vi "dfd_Validate SRate Quantizers for Code Gen.vi"(4 "FPGA?":bool=TRUE, 6 "LabVIEW?":bool=TRUE, 8 "error in (no error)":errorcluster, 11 "filter in":T1={"mSRate_Fs"=1.0, "mSRate_Version"="1.0", "mSRate_Comments"="", "mSRate_OrgCoef"={"type"=enum."Undefined", "gain"=1.0, "coef a (k)"=[], "coef b (v)"=[]}, "mSRate_CurCoef"={"type"=enum."Undefined", "gain"=1.0, "coef a (k)"=[], "coef b (v)"=[]}, "mSRate_Quantized?"=FALSE, "mSRate_QCoef"={"type"=enum."Undefined", "gain"=1.0, "coef a (k)"=[], "coef b (v)"=[]}, "mSRate_QSettings"=[], "mSRate_Order"=0, "mSRate_Scaling"={"mSRate_ScaleByPowerOf2?"=FALSE, "mSRate_ScaleType"=enum."No Norm"}} {"mSRate_QSettings"."source" items=["Coef a/k"=0, "Coef b/v"=7, "Input"=1, "Output"=2, "Multiplicand"=3, "Product"=4, "Sum"=5, "Delay"=6, "Gain"=8]}) -> (0 "error out":errorcluster, 3 "filter out":T1={"mSRate_Fs"=1.0, "mSRate_Version"="1.0", "mSRate_Comments"="", "mSRate_OrgCoef"={"type"=enum."Undefined", "gain"=1.0, "coef a (k)"=[], "coef b (v)"=[]}, "mSRate_CurCoef"={"type"=enum."Undefined", "gain"=1.0, "coef a (k)"=[], "coef b (v)"=[]}, "mSRate_Quantized?"=FALSE, "mSRate_QCoef"={"type"=enum."Undefined", "gain"=1.0, "coef a (k)"=[], "coef b (v)"=[]}, "mSRate_QSettings"=[], "mSRate_Order"=0, "mSRate_Scaling"={"mSRate_ScaleByPowerOf2?"=FALSE, "mSRate_ScaleType"=enum."No Norm"}} {"mSRate_QSettings"."source" items=["Coef a/k"=0, "Coef b/v"=7, "Input"=1, "Output"=2, "Multiplicand"=3, "Product"=4, "Sum"=5, "Delay"=6, "Gain"=8]})   [LabVIEW 2017, in "NI_DigFilterLicensed.lvlib"]
uses:
  <vilib>/addons/Digital Filter Design/NI_DigFilterLicensed.lvlib
  <vilib>/addons/Digital Filter Design/_Objects.llb/DFD Filter Obj.ctl
  <vilib>/addons/Digital Filter Design/_Objects.llb/DFD Filter Coef.ctl
  <vilib>/addons/Digital Filter Design/_Objects.llb/DFD Filter Structure Type Selector.ctl
  <vilib>/addons/Digital Filter Design/_Objects.llb/dfd_Internal Quantization Settings.ctl
  <vilib>/addons/Digital Filter Design/_Objects.llb/dfd_Internal Quantization Srcs.ctl
  <vilib>/addons/Digital Filter Design/_Objects.llb/DFD Coef Norm Type.ctl
  <vilib>/addons/Digital Filter Design/_Misc.llb/dfd_Error Handlers (Multiple).vi
  <vilib>/addons/Digital Filter Design/FilterLib.llb/dfd_Get Filter Coef Type (Filter IO).vi
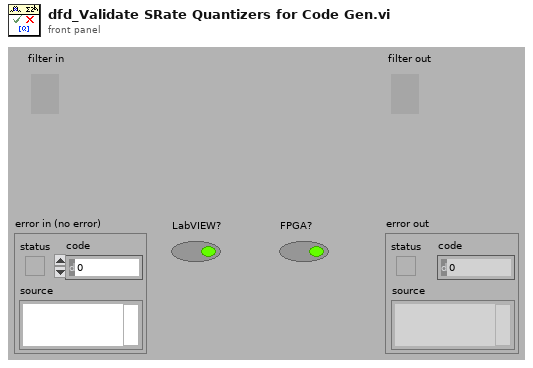
[diagram p1: front panel]
types:
  T1 = typedef "NI_DigFilterLicensed.lvlib/DFD Filter Obj.ctl" = cluster{"mSRate_Fs":dbl, "mSRate_Version":string, "mSRate_Comments":string, "mSRate_OrgCoef":T2, "mSRate_CurCoef":T2, "mSRate_Quantized?":bool, "mSRate_QCoef":T2, "mSRate_QSettings":T4[], "mSRate_Order":i32, "mSRate_Scaling":cluster{"mSRate_ScaleByPowerOf2?":bool, "mSRate_ScaleType":T6}}
  T2 = typedef "NI_DigFilterLicensed.lvlib/DFD Filter Coef.ctl" = cluster{"type":T3, "gain":dbl, "coef a (k)":dbl[], "coef b (v)":dbl[]}
  T3 = typedef "NI_DigFilterLicensed.lvlib/DFD Filter Structure Type Selector.ctl" = enum16{"Undefined", "FIR Direct Form", "FIR Direct Form Transposed", "FIR Symmetric", "FIR Antisymmetric", "IIR Direct Form I", "IIR Direct Form I Transposed", "IIR Direct Form II", "IIR Direct Form II Transposed", "IIR Cascaded Second Order Sections Form I", "IIR Cascaded Second Order Sections Form I Transposed", "IIR Cascaded Second Order Sections Form II", "IIR Cascaded Second Order Sections Form II Transposed", "Lattice Allpass (basic sections)", "Lattice Allpass (one multiplier sections)", "Lattice Allpass (normalized sections)", "Lattice AR (basic sections)", "Lattice AR (one multiplier sections)", "Lattice AR (normalized sections)", "Lattice MA (minimum phase)", "Lattice MA (maximum phase)", "Lattice ARMA (basic sections)", "Lattice ARMA (one multiplier sections)", "Lattice ARMA (normalized sections)"}
  T4 = typedef "NI_DigFilterLicensed.lvlib/dfd_Internal Quantization Settings.ctl" = cluster{"source":T5, "wl":i16, "iwl":i16, "overflow mode":enum16{"Saturation", "Wrap"}, "rounding mode":enum16{"Nearest", "Truncation"}, "signed?":bool}
  T5 = typedef "NI_DigFilterLicensed.lvlib/dfd_Internal Quantization Srcs.ctl" = u16
  T6 = typedef "NI_DigFilterLicensed.lvlib/DFD Coef Norm Type.ctl" = enum16{"No Norm", "Time Domain 1-Norm", "Time Domain 2-Norm", "Time Domain Inf-Norm"}
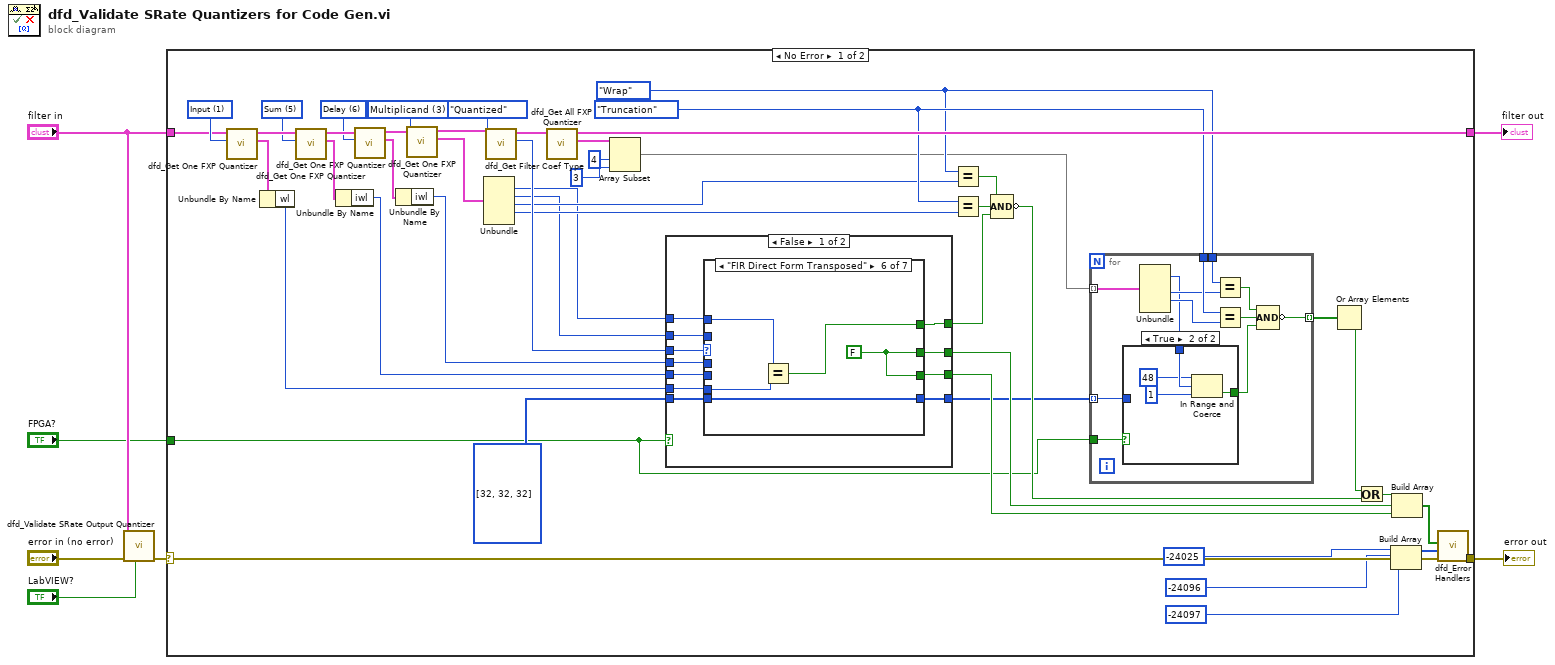
[diagram p0: block diagram]
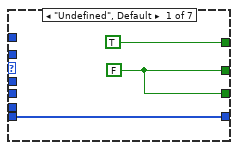
[diagram p2: hidden frame]
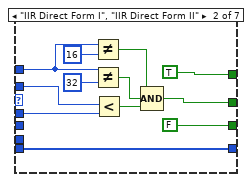
[diagram p3: hidden frame]
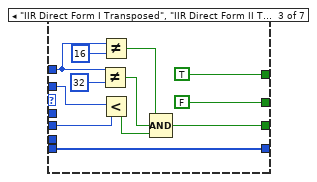
[diagram p4: hidden frame]
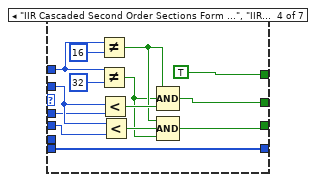
[diagram p5: hidden frame]
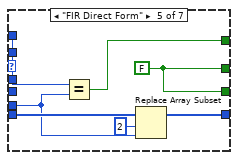
[diagram p6: hidden frame]
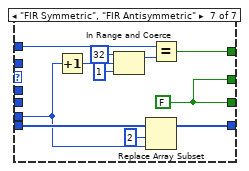
[diagram p7: hidden frame]
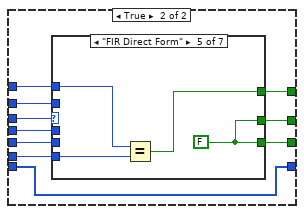
[diagram p8: hidden frame]
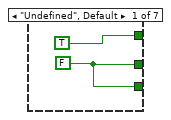
[diagram p9: hidden frame]
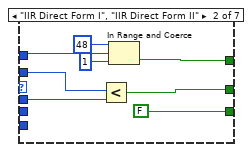
[diagram p10: hidden frame]
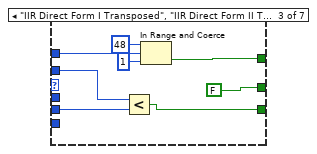
[diagram p11: hidden frame]
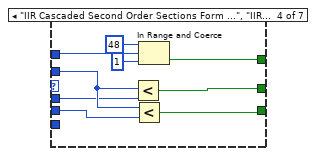
[diagram p12: hidden frame]
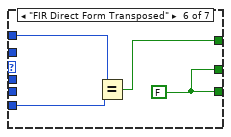
[diagram p13: hidden frame]
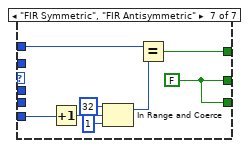
[diagram p14: hidden frame]
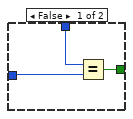
[diagram p15: hidden frame]
diagram:
  n1 = call <vilib>:"dfd_Validate SRate Output Quantizer.vi"("LabVIEW?"="LabVIEW?", "error in (no error)"="error in (no error)", "filter in"="filter in") -> ("error out"=w4:errorcluster)  [unwired: 8 out]
  n2 = case shown="No Error" w4 {
    selector: w4 -> [w43 w205]
    tunnel: [w56 w204] -> w7
    tunnel: "filter in" -> [w12 w204]
    tunnel: [w44 w205] -> w6
    tunnel: "FPGA?" -> [w8 _]
    frame No Error {
      w24 = T5 3 items=["Coef a/k"=0, "Coef b/v"=7, "Input"=1, "Output"=2, "Multiplicand"=3, "Product"=4, "Sum"=5, "Delay"=6, "Gain"=8] ("quantization source")
      w27 = T5 6 items=["Coef a/k"=0, "Coef b/v"=7, "Input"=1, "Output"=2, "Multiplicand"=3, "Product"=4, "Sum"=5, "Delay"=6, "Gain"=8] ("quantization source")
      w28 = T5 5 items=["Coef a/k"=0, "Coef b/v"=7, "Input"=1, "Output"=2, "Multiplicand"=3, "Product"=4, "Sum"=5, "Delay"=6, "Gain"=8] ("quantization source")
      w38 = enum16{"Nearest", "Truncation"}."Truncation" ("q_mode")
      w35 = enum16{"Saturation", "Wrap"}."Wrap" ("o_mode")
      w53 = T5 1 items=["Coef a/k"=0, "Coef b/v"=7, "Input"=1, "Output"=2, "Multiplicand"=3, "Product"=4, "Sum"=5, "Delay"=6, "Gain"=8] ("quantization source")
      n3 = call <vilib>:"dfd_Get One FXP Quantizer.vi"("quantization source"=w53, "filter in"=w12) -> ("quantization settings"=w55:T4, "filter out"=w34:T1)  [unwired: 1 in, 7 out]
      n4 = Unbundle By Name(w55) -> ("wl"=w50:i16)
      n5 = call <vilib>:"dfd_Get One FXP Quantizer.vi"("quantization source"=w28, "filter in"=w34) -> ("quantization settings"=w26:T4, "filter out"=w33:T1)  [unwired: 1 in, 7 out]
      n6 = Unbundle By Name(w26) -> ("iwl"=w20:i16)
      n7 = call <vilib>:"dfd_Get One FXP Quantizer.vi"("quantization source"=w27, "filter in"=w33) -> ("quantization settings"=w25:T4, "filter out"=w32:T1)  [unwired: 1 in, 7 out]
      n8 = Unbundle By Name(w25) -> ("iwl"=w21:i16)
      n9 = call <vilib>:"dfd_Get One FXP Quantizer.vi"("quantization source"=w24, "filter in"=w32) -> ("quantization settings"=w30:T4, "filter out"=w31:T1)  [unwired: 1 in, 7 out]
      n10 = Unbundle(w30) -> ("wl"=w22:i16, "iwl"=w23:i16, "overflow mode"=w29:enum16{"Saturation", "Wrap"}, "rounding mode"=w39:enum16{"Nearest", "Truncation"})  [unwired: 2 out]
      n11 = call-poly <vilib>:"dfd_Get Filter Coef Type.vi"("coef source"=enum16{"Original", "Current", "Quantized"}."Quantized", "filter in"=w31) -> ("type"=w51:T3, "filter out"=w52:T1)  [unwired: 2 in, 6 out]
      n12 = call <vilib>:"dfd_Get All FXP Quantizer.vi"("filter in"=w52) -> ("quantization settings"=w49:T4[], "filter out"=w56:T1)  [unwired: 1 in, 8 out]
      n13 = Array Subset(array=w49, index=4, length=3) -> (w11:T4[])
      n14 = case shown="False" w8 {
        tunnel: w51 -> [w65 w141]
        tunnel: w50 -> [w62 w140]
        tunnel: [w61 w139] -> w37
        tunnel: w23 -> [w66 w138]
        tunnel: w22 -> [w67 w137]
        tunnel: w21 -> [w64 w136]
        tunnel: w20 -> [w63 w135]
        tunnel: [w60 w134] -> w18
        tunnel: [w59 w133] -> w17
        tunnel: i16[] [32, 32, 32] -> [w58 w132]
        tunnel: [w57 w132] -> w9
        frame False {
          n15 = case shown="\"FIR Direct Form Transposed\"" w65 {
            tunnel: w62 -> [_ _ _ _ w110 w120 w121]
            tunnel: [TRUE TRUE TRUE TRUE w115 w118 w125] -> w61
            tunnel: w67 -> [_ w75 w87 w98 w114 w119 w127]
            tunnel: w66 -> [_ w81 w93 w103 _ _ _]
            tunnel: w64 -> [_ w80 _ w102 _ _ _]
            tunnel: w63 -> [_ _ w92 w101 _ _ _]
            tunnel: [w69 w77 FALSE w105 w113 w117 w126] -> w60
            tunnel: [w69 FALSE w89 w100 w113 w117 w126] -> w59
            tunnel: w58 -> [w68 w71 w83 w95 w111 w116 w122]
            tunnel: [w68 w71 w83 w95 w109 w116 w123] -> w57
            frame "Undefined", Default {
              w69 = FALSE
            }
            frame "IIR Direct Form I", "IIR Direct Form II" {
              n16 = Not Equal?(x=w75, y=i16 16) -> (x != y?=w73:bool)
              n17 = Not Equal?(x=w75, y=i16 32) -> (x != y?=w72:bool)
              n18 = Less?(x=w81, y=w80) -> (x < y?=w79:bool)
              n19 = Compound Arithmetic op=AND(w73, w72, w79) -> (w77:bool)
            }
            frame "IIR Direct Form I Transposed", "IIR Direct Form II Transposed", "IIR Cascaded Second Order Sections Form I Transposed", "IIR Cascaded Second Order Sections Form II Transposed", "Lattice Allpass (one multiplier sections)", "Lattice AR (one multiplier sections)", "Lattice ARMA (one multiplier sections)" {
              n20 = Not Equal?(x=w87, y=i16 32) -> (x != y?=w85:bool)
              n21 = Not Equal?(x=w87, y=i16 16) -> (x != y?=w86:bool)
              n22 = Less?(x=w93, y=w92) -> (x < y?=w84:bool)
              n23 = Compound Arithmetic op=AND(w86, w85, w84) -> (w89:bool)
            }
            frame "IIR Cascaded Second Order Sections Form I", "IIR Cascaded Second Order Sections Form II", "Lattice Allpass (basic sections)", "Lattice Allpass (normalized sections)", "Lattice AR (basic sections)", "Lattice AR (normalized sections)".."Lattice ARMA (basic sections)", "Lattice ARMA (normalized sections)" {
              n24 = Not Equal?(x=w98, y=i16 16) -> (x != y?=w97:bool)
              n25 = Not Equal?(x=w98, y=i16 32) -> (x != y?=w96:bool)
              n26 = Less?(x=w103, y=w102) -> (x < y?=w107:bool)
              n27 = Less?(x=w103, y=w101) -> (x < y?=w104:bool)
              n28 = Compound Arithmetic op=AND(w97, w96, w107) -> (w105:bool)
              n29 = Compound Arithmetic op=AND(w97, w104, w96) -> (w100:bool)
            }
            frame "FIR Direct Form" {
              w113 = FALSE
              n30 = Equal?(x=w114, y=w110) -> (x = y?=w115:bool)
              n31 = Replace Array Subset(array=w111, new element=w110, index=2) -> (w109:i16[])
            }
            frame "FIR Direct Form Transposed" {
              w117 = FALSE
              n32 = Equal?(x=w119, y=w120) -> (x = y?=w118:bool)
            }
            frame "FIR Symmetric", "FIR Antisymmetric" {
              w126 = FALSE
              n33 = Increment(x=w121) -> (x+1=w131:i16)
              n34 = In Range and Coerce(upper limit=i16 32, x=w131, lower limit=i16 1) -> (coerced(x)=w128:i16)  [unwired: 1 out]
              n35 = Replace Array Subset(array=w122, new element=w121, index=2) -> (w123:i16[])
              n36 = Equal?(x=w127, y=w128) -> (x = y?=w125:bool)
            }
          }
        }
        frame True {
          n37 = case shown="\"FIR Direct Form\"" w141 {
            tunnel: w140 -> [_ _ _ _ w172 w176 w184]
            tunnel: [TRUE w144 w153 w162 w171 w174 w177] -> w139
            tunnel: w137 -> [_ w146 w154 w163 w170 w175 w179]
            tunnel: w138 -> [_ w151 w159 w168 _ _ _]
            tunnel: w136 -> [_ w150 _ w167 _ _ _]
            tunnel: w135 -> [_ _ w158 w166 _ _ _]
            tunnel: [w142 w145 FALSE w161 w169 w173 w178] -> w134
            tunnel: [w142 FALSE w152 w160 w169 w173 w178] -> w133
            frame "Undefined", Default {
              w142 = FALSE
            }
            frame "IIR Direct Form I", "IIR Direct Form II" {
              n38 = Less?(x=w151, y=w150) -> (x < y?=w145:bool)
              n39 = In Range and Coerce(upper limit=i16 48, x=w146, lower limit=i16 1) -> (In Range?=w144:bool)  [unwired: 1 out]
            }
            frame "IIR Direct Form I Transposed", "IIR Direct Form II Transposed", "IIR Cascaded Second Order Sections Form I Transposed", "IIR Cascaded Second Order Sections Form II Transposed", "Lattice Allpass (one multiplier sections)", "Lattice AR (one multiplier sections)", "Lattice ARMA (one multiplier sections)" {
              n40 = Less?(x=w159, y=w158) -> (x < y?=w152:bool)
              n41 = In Range and Coerce(upper limit=i16 48, x=w154, lower limit=i16 1) -> (In Range?=w153:bool)  [unwired: 1 out]
            }
            frame "IIR Cascaded Second Order Sections Form I", "IIR Cascaded Second Order Sections Form II", "Lattice Allpass (basic sections)", "Lattice Allpass (normalized sections)", "Lattice AR (basic sections)", "Lattice AR (normalized sections)".."Lattice ARMA (basic sections)", "Lattice ARMA (normalized sections)" {
              n42 = Less?(x=w168, y=w167) -> (x < y?=w161:bool)
              n43 = Less?(x=w168, y=w166) -> (x < y?=w160:bool)
              n44 = In Range and Coerce(upper limit=i16 48, x=w163, lower limit=i16 1) -> (In Range?=w162:bool)  [unwired: 1 out]
            }
            frame "FIR Direct Form" {
              w169 = FALSE
              n45 = Equal?(x=w170, y=w172) -> (x = y?=w171:bool)
            }
            frame "FIR Direct Form Transposed" {
              w173 = FALSE
              n46 = Equal?(x=w175, y=w176) -> (x = y?=w174:bool)
            }
            frame "FIR Symmetric", "FIR Antisymmetric" {
              w178 = FALSE
              n47 = Increment(x=w184) -> (x+1=w183:i16)
              n48 = In Range and Coerce(upper limit=i16 32, x=w183, lower limit=i16 1) -> (coerced(x)=w180:i16)  [unwired: 1 out]
              n49 = Equal?(x=w179, y=w180) -> (x = y?=w177:bool)
            }
          }
        }
      }
      n50 = Equal?(x=w35, y=w29) -> (x = y?=w41:bool)
      n51 = Equal?(x=w38, y=w39) -> (x = y?=w40:bool)
      n52 = Compound Arithmetic op=AND(w41, w40, w37) -> (invert w36:bool)
      n53 = for {
        tunnel: w11 -> [w196] mode=indexing
        tunnel: w38 -> [w194]
        tunnel: w35 -> [w192]
        tunnel: [w189] -> w46 mode=indexing
        tunnel: w9 -> [w186] mode=indexing
        tunnel: w8 -> [w185]
        n54 = Unbundle(w196) -> ("wl"=w188:i16, "overflow mode"=w193:enum16{"Saturation", "Wrap"}, "rounding mode"=w195:enum16{"Nearest", "Truncation"})  [unwired: 3 out]
        n55 = case shown="True" w185 {
          tunnel: w188 -> [w199 w203]
          tunnel: [w198 w200] -> w187
          tunnel: w186 -> [w197 _]
          frame False {
            n56 = Equal?(x=w199, y=w197) -> (x = y?=w198:bool)
          }
          frame True {
            n57 = In Range and Coerce(upper limit=i16 48, x=w203, lower limit=i16 1) -> (In Range?=w200:bool)  [unwired: 1 out]
          }
        }
        n58 = Equal?(x=w192, y=w193) -> (x = y?=w190:bool)
        n59 = Equal?(x=w194, y=w195) -> (x = y?=w191:bool)
        n60 = Compound Arithmetic op=AND(w190, w191, w187) -> (invert w189:bool)
      }
      n61 = Or Array Elements(Boolean array=w46) -> (logical OR=w42:bool)
      n62 = Or(x=w42, y=w36) -> (x .or. y?=w13:bool)
      n63 = Build Array(-24025 ("ERR_CODE_UNSUPPORT_MODEL"), -24096 ("ERR_MULT_LT_DELAY"), -24097 ("ERR_MULT_LT_SUM")) -> (w16:i32[])
      n64 = Build Array(w13, w18, w17) -> (w19:bool[])
      n65 = call-poly <vilib>:"dfd_Error Handlers.vi"("error in (no error)"=w43, "error sources"=w16, "condition failed?"=w19) -> ("error out"=w44:errorcluster)  [unwired: 8 out]
    }
    frame Error {
    }
  }
  "filter out" <- w7
  "error out" <- w6
